vi "fft2sym.vi"(1 "Number of Subcarriers":i32, 2 "Time domain In":cdb[](array[numeric])) -> (0 "Parallel Symbole out 2":cdb[](array[numeric]))   [LabVIEW 2013]
uses:
  <vilib>/Analysis/2dsp.llb/Complex FFT.vi
  <vilib>/Analysis/NI_AALPro.lvlib
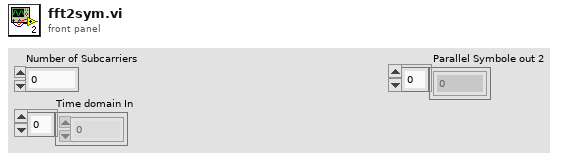
[diagram p1: front panel]
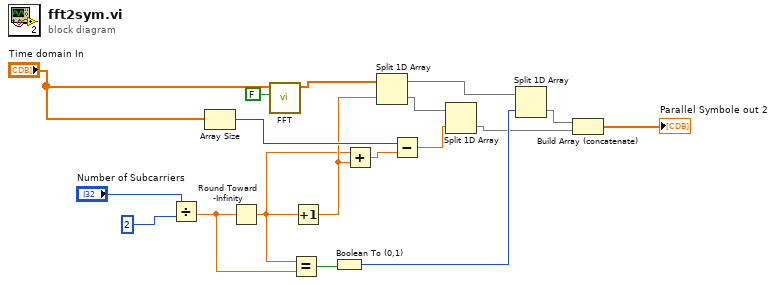
[diagram p0: block diagram]
diagram:
  n1 = Divide(x="Number of Subcarriers", y=2) -> (x/y=w10:dbl)
  n2 = Array Size(array="Time domain In") -> (size(s)=w13:i32)
  n3 = Round Toward -Infinity(1:w10) -> (0:w11:dbl)
  n4 = call-poly <vilib>:"FFT.vi"("shift?"=FALSE, "X"="Time domain In") -> ("FFT {X}"=w14:cdb[])  [unwired: 8 in, 1 out]
  n5 = Equal?(x=w11, y=w10) -> (x = y?=w17:bool)
  n6 = Increment(x=w11) -> (x+1=w12:dbl)
  n7 = Boolean To (0,1)(Boolean=w17) -> (0, 1=w7:i16)
  n8 = Add(x=w11, y=w12) -> (x+y=w18:dbl)
  n9 = Split 1D Array(array=w14, index=w12) -> (first subarray=w6:cdb[], second subarray=w16:cdb[])
  n10 = Subtract(x=w13, y=w18) -> (x-y=w5:dbl)
  n11 = Split 1D Array(array=w16, index=w5) -> (second subarray=w3:cdb[])  [unwired: 1 out]
  n12 = Split 1D Array(array=w6, index=w7) -> (second subarray=w4:cdb[])  [unwired: 1 out]
  n13 = Build Array (concatenate)(w4, w3) -> (→"Parallel Symbole out 2":cdb[])
